vi "Execute.vi"(8 "error in (no error)":errorcluster, 10 "Execution":refnum<data-value>, 11 "VIStep in":refnum<class "CallVIStep.lvclass">) -> (0 "error out":errorcluster, 1 "Output Values":cluster{"Name":string, "Variant Data":variant}[](array[cluster]), 3 "VIStep out":refnum<class "CallVIStep.lvclass">)   [LabVIEW 2015, in "CallVIStep.lvclass"]
uses:
  CallVIStep.lvclass
  Execution.lvclass
  VI_EXECUTE_STATE.ctl
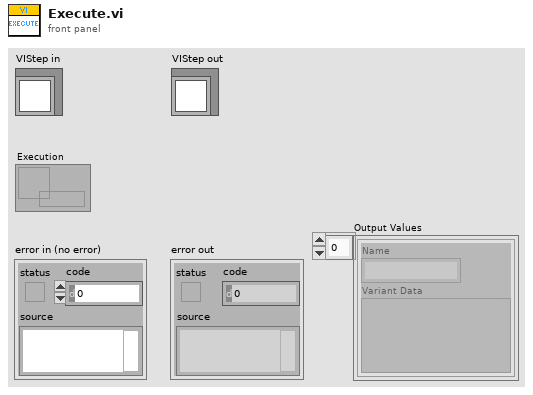
[diagram p1: front panel]
types:
  T1 = typedef "CallVIStep.lvclass/VI_EXECUTE_STATE.ctl" = enum16{"OPEN_VI", "INJECT_CLASS_INSTANCE", "SET_INPUTS", "SHOW_PANEL", " RUN", "UPDATE_CLASS_INSTANCE", "GET_OUTPUTS", "CLOSE_PANEL", "CLOSE_VI", "END"}
  T2 = enum32{"Invalid", "Standard", "Closed", "Hidden", "Minimized", "Maximized"}
  T3 = typedef "CallVIStep.lvclass/VI Input Typedef.ctl" = cluster{"Label":string, "Input Type":T4, "Type String":i16[], "Data String":string, "Variable Name":string}
  T4 = typedef "CallVIStep.lvclass/VI Input Type Typedef.ctl" = enum16{"Default", "Value", "Variable"}
  T5 = typedef "Step.lvclass/STEP_OUTPUT.ctl" = cluster{"Label":string, "Name":string, "Data Type":T6, "Check Type":T7, "String Limit":string, "Lower Limit":dbl, "Upper Limit":dbl, "Boolean Limit":bool, "Ignore Case":bool, "Variable Name 1":string, "Limit Value Type 1":T8, "Variable Name 2":string, "Limit Value Type 2":T8}
  T6 = typedef "Step.lvclass/OUTPUT_DATA_TYPE.ctl" = enum16{"Boolean", "String", "Numeric", "Other"}
  T7 = typedef "Step.lvclass/OUTPUT_CHECK_TYPE.ctl" = enum16{"INVALID", "DO_NOT_CHECK", "RECORD", "VARIABLE", "EQUAL", "NOT_EQUAL", "STR_CONTAINS", "STR_START_WITH", "STR_END_WITH", "STR_REGEX_MATCH", "NUM_GT", "NUM_LT", "NUM_GE", "NUM_LE", "NUM_RANGE", "NUM_RANGE_BDY"}
  T8 = typedef "Step.lvclass/OUTPUT_VALUE_TYPE.ctl" = enum16{"Constant", "Variable"}
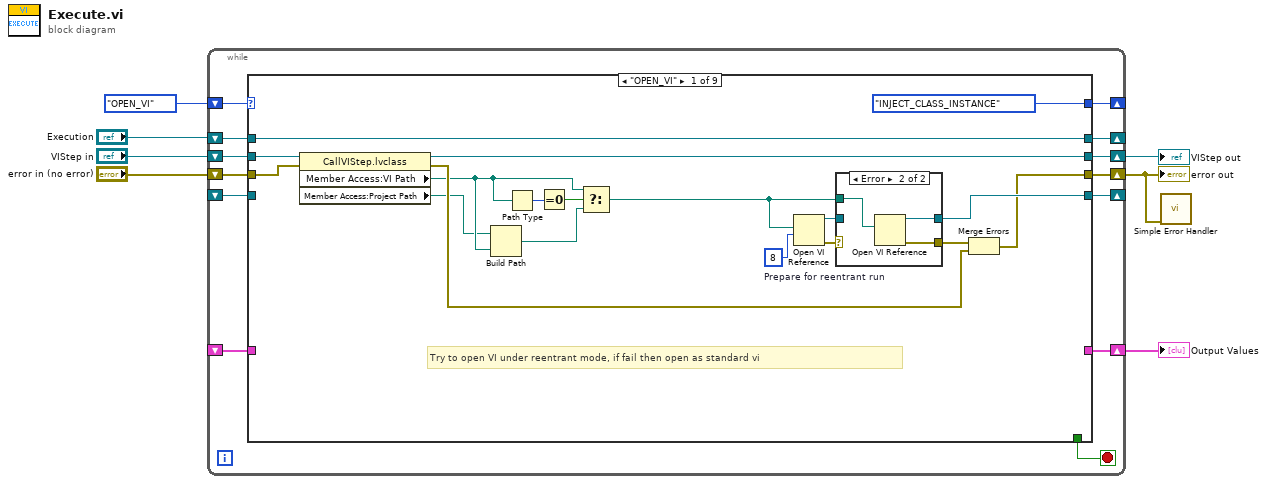
[diagram p0: block diagram]
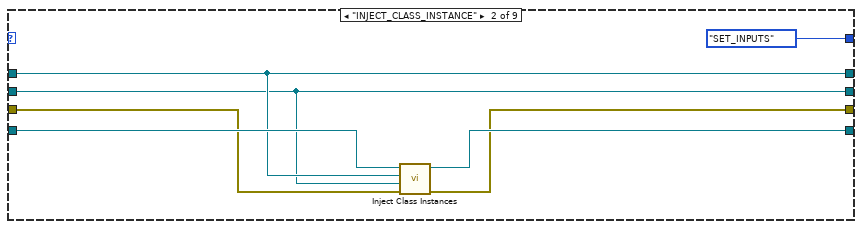
[diagram p3: hidden frame]
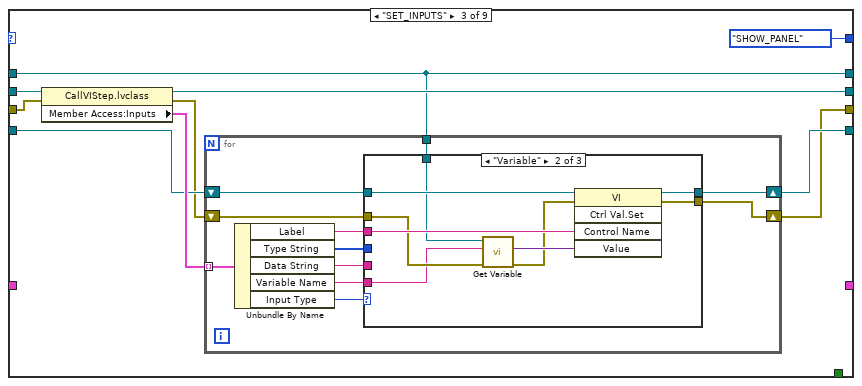
[diagram p4: hidden frame]
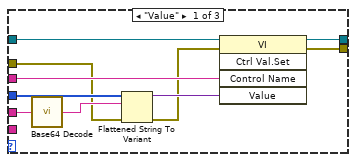
[diagram p5: hidden frame]
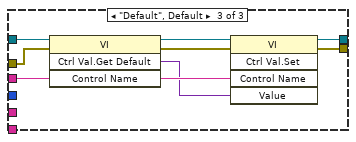
[diagram p6: hidden frame]
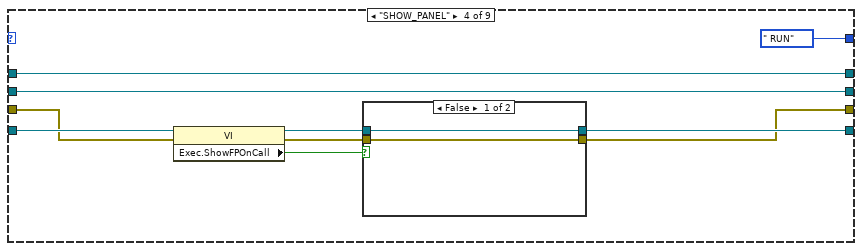
[diagram p7: hidden frame]
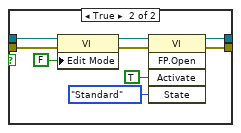
[diagram p8: hidden frame]
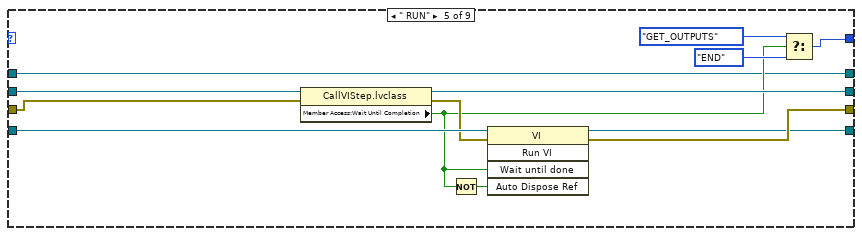
[diagram p9: hidden frame]
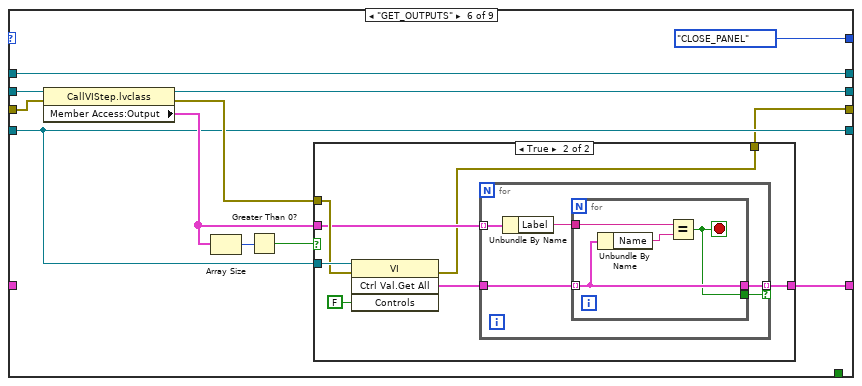
[diagram p10: hidden frame]
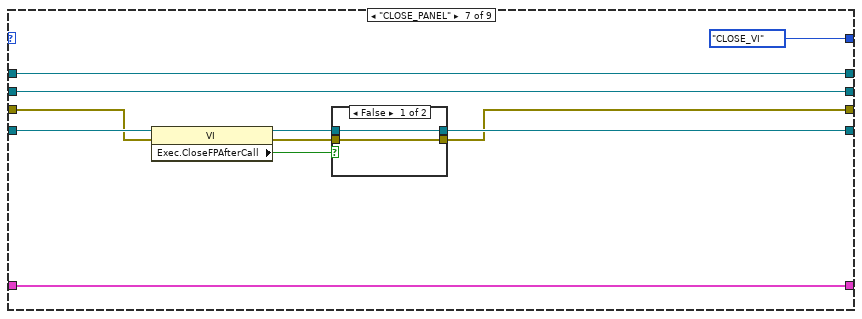
[diagram p12: hidden frame]
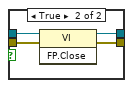
[diagram p13: hidden frame]
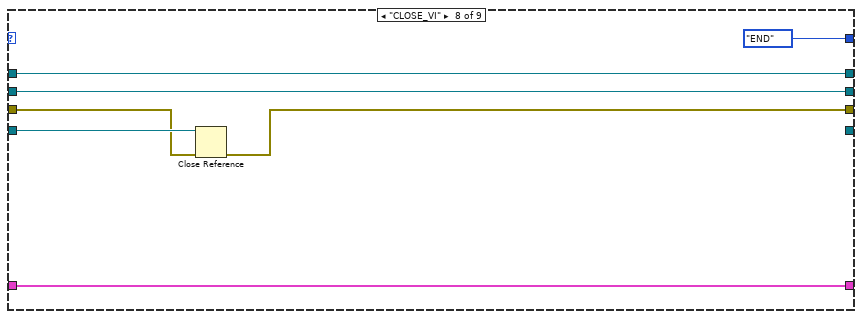
[diagram p14: hidden frame]
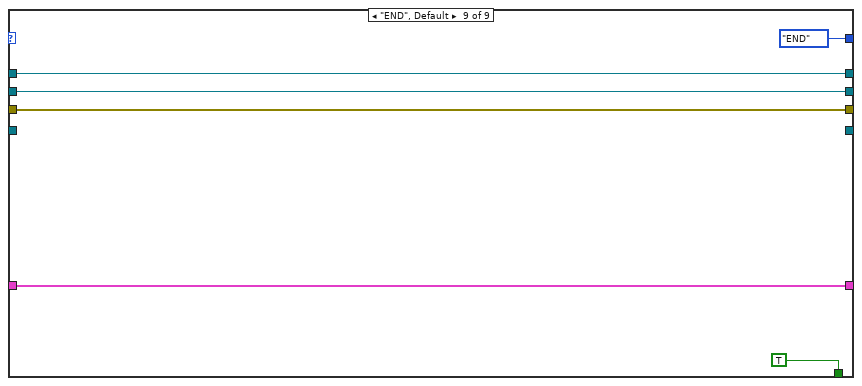
[diagram p15: hidden frame]
diagram:
  n1 = while {
    shift-right: [w14] -> w4
    shift-left: "VIStep in" -> [w19]
    shift-right: [w16] -> w2
    shift-left: "error in (no error)" -> [w18]
    shift-right: [w17] -> _
    shift-left: _ -> [w15]
    shift-right: [w13] -> _
    shift-left: VI_EXECUTE_STATE."OPEN_VI" -> [w20]
    shift-right: [w11] -> w3
    shift-left: _ -> [w10]
    shift-right: [w9] -> _
    shift-left: "Execution" -> [w8]
    stop <- w12 stop-if-true
    n2 = case shown="\"OPEN_VI\"" w20 {
      tunnel: w19 -> [w38 w44 w60 w108 w132 w143 w167 w182 w189]
      tunnel: w18 -> [w37 w46 w55 w106 w131 w142 w168 w184 w190]
      tunnel: [w31 w48 w58 w102 w126 w136 w166 _ _] -> w17
      tunnel: [w28 w47 w57 w101 w127 w135 w165 w183 w190] -> w16
      tunnel: w15 -> [_ w49 w53 w107 w130 w136 w169 w185 _]
      tunnel: [w36 w44 w56 w108 w128 w134 w167 w182 w189] -> w14
      tunnel: [VI_EXECUTE_STATE."INJECT_CLASS_INSTANCE" VI_EXECUTE_STATE."SET_INPUTS" VI_EXECUTE_STATE."SHOW_PANEL" VI_EXECUTE_STATE." RUN" w123 VI_EXECUTE_STATE."CLOSE_PANEL" VI_EXECUTE_STATE."CLOSE_VI" VI_EXECUTE_STATE."END" VI_EXECUTE_STATE."END"] -> w13
      tunnel: [_ _ _ _ _ _ _ _ TRUE] -> w12
      tunnel: [_ _ _ _ _ w137 w163 w180 w187] -> w11
      tunnel: w10 -> [_ _ _ _ _ _ w163 w180 w187]
      tunnel: w8 -> [w23 w45 w51 w99 w120 w133 w162 w179 w186]
      tunnel: [w23 w45 w51 w99 w120 w133 w162 w179 w186] -> w9
      frame "OPEN_VI" {
        w34 = 8  # Prepare for reentrant run
        # "Try to open VI under reentrant mode, if fail then open as standard vi"
        n3 = property class="CallVIStep.lvclass"(reference=w38, error in=w37) -> (reference out=w36:refnum<class "CallVIStep.lvclass">, error out=w29:errorcluster, "Member Access:VI Path"=w25:path, "Member Access:Project Path"=w21:path)
        n4 = Build Path(base path=w21, name or relative path=w25) -> (appended path=w24:path)
        n5 = Path Type(1:w25) -> (0:w27:i16)
        n6 = Equal To 0?(x=w27) -> (x = 0?=w26:bool)
        n7 = Select(t=w25, s=w26, f=w24) -> (s? t:f=w22:path)
        n8 = Open VI Reference(vi path=w22, options=w34) -> (vi reference=w32:refnum<vi>, error out=w33:errorcluster)  [unwired: 4 in]
        n9 = case shown="Error" w33 {
          selector: w33 -> [w39 _]
          tunnel: w32 -> [w40 _]
          tunnel: w22 -> [_ w43]
          tunnel: [w39 w42] -> w30
          tunnel: [w40 w41] -> w31
          frame No Error {
          }
          frame Error {
            n10 = Open VI Reference(vi path=w43) -> (vi reference=w41:refnum<vi>, error out=w42:errorcluster)  [unwired: 5 in]
          }
        }
        n11 = Merge Errors(w30, w29) -> (w28:errorcluster)
      }
      frame "INJECT_CLASS_INSTANCE" {
        n12 = call "Inject Class Instances.vi"("error in (no error)"=w46, "Step in"=w44, "Execution in"=w45, "VI Refnum in"=w49) -> ("error out"=w47:errorcluster, "VI Refnum out"=w48:refnum<vi>)  [unwired: 6 in]
      }
      frame "SET_INPUTS" {
        n13 = property class="CallVIStep.lvclass"(reference=w60, error in=w55) -> (reference out=w56:refnum<class "CallVIStep.lvclass">, error out=w52:errorcluster, "Member Access:Inputs"=w59:T3[])
        n14 = for {
          tunnel: w59 -> [w71] mode=indexing
          shift-right: [w64] -> w57
          shift-left: w52 -> [w65]
          shift-right: [w66] -> w58
          shift-left: w53 -> [w68]
          tunnel: w51 -> [w61]
          n15 = Unbundle By Name(w71) -> ("Label"=w67:string, "Type String"=w69:i16[], "Data String"=w70:string, "Variable Name"=w62:string, "Input Type"=w63:T4)
          n16 = case shown="\"Variable\"" w63 {
            tunnel: w70 -> [w81 _ _]
            tunnel: w69 -> [w79 _ _]
            tunnel: w68 -> [w78 w90 w98]
            tunnel: w67 -> [w77 w89 w92]
            tunnel: [w75 w88 w95] -> w66
            tunnel: w65 -> [w74 w84 w97]
            tunnel: [w72 w87 w93] -> w64
            tunnel: w62 -> [_ w82 _]
            tunnel: w61 -> [_ w86 _]
            frame "Value" {
              n17 = call "Base64 Decode.vi"("base64 string"=w81) -> ("normal string"=w80:string)
              n18 = Flattened String To Variant(4:w74, 6:w80, 7:w79) -> (0:w73:errorcluster, 3:w76:variant)
              n19 = invoke class="VI" method="Ctrl Val.Set"(reference=w78, error in=w73, "Control Name"=w77, "Value"=w76) -> (reference out=w75:refnum<vi>, error out=w72:errorcluster)  [unwired: 1 in, 3 out]
            }
            frame "Variable" {
              n20 = call "Get Variable.vi"("error in (no error)"=w84, "Name"=w82, "Execution in"=w86) -> ("error out"=w83:errorcluster, "Value"=w85:variant)  [unwired: 6 in, 1 out]
              n21 = invoke class="VI" method="Ctrl Val.Set"(reference=w90, error in=w83, "Control Name"=w89, "Value"=w85) -> (reference out=w88:refnum<vi>, error out=w87:errorcluster)  [unwired: 1 in, 3 out]
            }
            frame "Default", Default {
              n22 = invoke class="VI" method="Ctrl Val.Get Default"(reference=w98, error in=w97, "Control Name"=w92) -> (reference out=w96:refnum<vi>, error out=w94:errorcluster, "Ctrl Val.Get Default"=w91:variant)  [unwired: 1 in, 1 out]
              n23 = invoke class="VI" method="Ctrl Val.Set"(reference=w96, error in=w94, "Control Name"=w92, "Value"=w91) -> (reference out=w95:refnum<vi>, error out=w93:errorcluster)  [unwired: 1 in, 3 out]
            }
          }
        }
      }
      frame "SHOW_PANEL" {
        n24 = property class="VI"(reference=w107, error in=w106) -> (reference out=w104:refnum<vi>, error out=w105:errorcluster, "Exec.ShowFPOnCall"=w103:bool)
        n25 = case shown="False" w103 {
          tunnel: w105 -> [w110 w113]
          tunnel: w104 -> [w109 w115]
          tunnel: [w110 w117] -> w101
          tunnel: [w109 w116] -> w102
          frame False {
          }
          frame True {
            n26 = property class="VI"(reference=w115, error in=w113, "Edit Mode"=FALSE ("Edit Mode On Open")) -> (reference out=w112:refnum<vi>, error out=w111:errorcluster)
            n27 = invoke class="VI" method="FP.Open"(reference=w112, error in=w111, "Activate"=TRUE ("Activate?"), "State"=T2."Standard") -> (reference out=w116:refnum<vi>, error out=w117:errorcluster)  [unwired: 1 in, 3 out]
          }
        }
      }
      frame " RUN" {
        n28 = property class="CallVIStep.lvclass"(reference=w132, error in=w131) -> (reference out=w128:refnum<class "CallVIStep.lvclass">, error out=w129:errorcluster, "Member Access:Wait Until Completion"=w122:bool)
        n29 = Not(x=w122) -> (.not. x?=w121:bool)
        n30 = invoke class="VI" method="Run VI"(reference=w130, error in=w129, "Wait until done"=w122, "Auto Dispose Ref"=w121) -> (reference out=w126:refnum<vi>, error out=w127:errorcluster)  [unwired: 1 in, 3 out]
        n31 = Select(t=VI_EXECUTE_STATE."GET_OUTPUTS", s=w122, f=VI_EXECUTE_STATE."END") -> (s? t:f=w123:T1)
      }
      frame "GET_OUTPUTS" {
        n32 = property class="CallVIStep.lvclass"(reference=w143, error in=w142) -> (reference out=w134:refnum<class "CallVIStep.lvclass">, error out=w138:errorcluster, "Member Access:Output"=w139:T5[])
        n33 = Array Size(array=w139) -> (size(s)=w141:i32)
        n34 = Greater Than 0?(x=w141) -> (x > 0?=w140:bool)
        n35 = case shown="True" w140 {
          tunnel: w136 -> [_ w152]
          tunnel: w139 -> [_ w149]
          tunnel: w138 -> [w145 w150]
          tunnel: [_ w147] -> w137
          tunnel: [w145 w146] -> w135
          frame False {
          }
          frame True {
            n36 = invoke class="VI" method="Ctrl Val.Get All"(reference=w152, error in=w150, "Controls"=FALSE) -> (error out=w146:errorcluster, "Get All Control Values Variant"=w148:cluster{"Name":string, "Variant Data":variant}[])  [unwired: 1 in, 2 out]
            n37 = for {
              tunnel: w149 -> [w157] mode=indexing
              tunnel: w148 -> [w156]
              tunnel: [w154] -> w147 mode=indexing if=w153
              n38 = Unbundle By Name(w157) -> ("Label"=w155:string)
              n39 = for {
                tunnel: w156 -> [w159] mode=indexing
                tunnel: w155 -> [w160]
                tunnel: [w159] -> w154
                tunnel: [w158] -> w153
                stop <- w158 stop-if-true
                n40 = Unbundle By Name(w159) -> ("Name"=w161:string)
                n41 = Equal?(x=w160, y=w161) -> (x = y?=w158:bool)
              }
            }
          }
        }
      }
      frame "CLOSE_PANEL" {
        n42 = property class="VI"(reference=w169, error in=w168) -> (reference out=w171:refnum<vi>, error out=w172:errorcluster, "Exec.CloseFPAfterCall"=w170:bool)
        n43 = case shown="False" w170 {
          tunnel: w171 -> [w174 w178]
          tunnel: w172 -> [w173 w177]
          tunnel: [w174 w176] -> w166
          tunnel: [w173 w175] -> w165
          frame False {
          }
          frame True {
            n44 = invoke class="VI" method="FP.Close"(reference=w178, error in=w177) -> (reference out=w176:refnum<vi>, error out=w175:errorcluster)  [unwired: 1 in, 1 out]
          }
        }
      }
      frame "CLOSE_VI" {
        n45 = Close Reference(reference=w185, error in (no error)=w184) -> (error out=w183:errorcluster)
      }
      frame "END", Default {
      }
    }
  }
  "error out" <- w2
  "VIStep out" <- w4
  "Output Values" <- w3
  n46 = call <vilib>:"Simple Error Handler.vi"("error in (no error)"=w2) -> ()  [unwired: 4 in, 5 out]
